vi "Sagar C V Basic gates using NAND Gate.vi"() -> ()   [LabVIEW 2018]
panel:
  out "NOT GATE USING NAND GATE":bool
  out "OR GATE USING NAND GATE":bool
  out "AND GATE USING NAND GATE":bool
  in  "E":bool
  in  "D":bool
  in  "C":bool
  in  "B":bool
  in  "A":bool
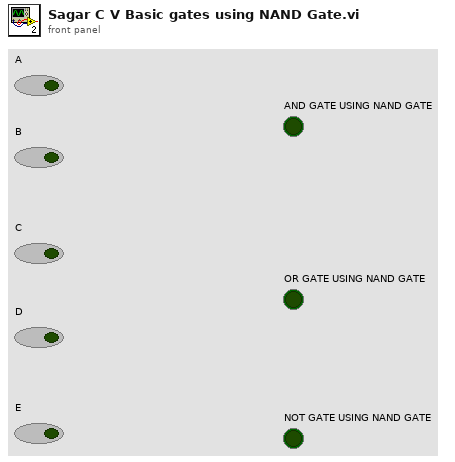
[diagram p1: front panel]
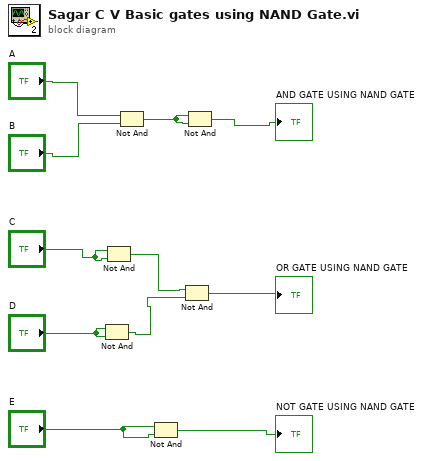
[diagram p0: block diagram]
diagram:
  n1 = Not And(1:"D", 2:"D") -> (0:w5:bool)
  n2 = Not And(1:"C", 2:"C") -> (0:w6:bool)
  n3 = Not And(1:"B", 2:"A") -> (0:w10:bool)
  n4 = Not And(1:"E", 2:"E") -> (0:→"NOT GATE USING NAND GATE":bool)
  n5 = Not And(1:w5, 2:w6) -> (0:→"OR GATE USING NAND GATE":bool)
  n6 = Not And(1:w10, 2:w10) -> (0:→"AND GATE USING NAND GATE":bool)
